vi "Detect QR Code.vi"() -> ()   [LabVIEW 2020, in "examples.lvlib"]
doc: "Demonstrate the QR Code Encoder and the WeChat QR Code Detector."
uses:
  examples.lvlib
  feature_detection/WeChat QR Code Detector/Detection.ctl
  common/Image Points Quad (Float).ctl
  common/Image Point (Float).ctl
  <vilib>/Utility/sysdir.llb/System Directory Type.ctl
  feature_detection/QR Code Encoder/Correction Levels.ctl
  feature_detection/QR Code Encoder/QR Code Encoder.lvclass/QR Code Encoder.ctl
  feature_detection/WeChat QR Code Detector/WeChat QR Code Detector.lvclass/WeChat QR Code Detector.ctl
  image/ARGB Colour.ctl
  feature_detection/QR Code Encoder/Create (Single).vi
  feature_detection/QR Code Encoder/Encode (Single).vi
  image/New Image (ARGB Array).vi
  feature_detection/WeChat QR Code Detector/Detect and Decode Multiple (ARGB).vi
  image/Draw Poly Lines (ARGB).vi
  image/Draw Image to Picture (ARGB).vi
  feature_detection/QR Code Encoder/CreateCore.vi
  feature_detection/QR Code Encoder/EncodeSingleCore.vi
  feature_detection/WeChat QR Code Detector/Detect and Decode Multiple (ARGB).vi/947807d6-cf22-42cc-b024-3c0d53b5d2ed.vi
  image/ARGB Colour to U32 Pixel Value.vi
  image/Draw Poly Lines (ARGB).vi/f4fe866f-059f-471d-887d-2797bd4b3b13.vi
  image/Draw Image to Picture (ARGB).vi/8cd07b1b-062e-4fe4-9e87-2eb3dc89fe0e.vi
  <vilib>/Utility/error.llb/Error Cluster From Error Code.vi
  feature_detection/WeChat QR Code Detector/Create (Model Files Folder).vi
  feature_detection/QR Code Encoder/QR Code Encoder.lvclass
  image/image.lvlib
  feature_detection/WeChat QR Code Detector/WeChat QR Code Detector.lvclass
  common/common.lvlib
panel:
  out "Detections":T1[](array[typedef])
  out "Picture":picture
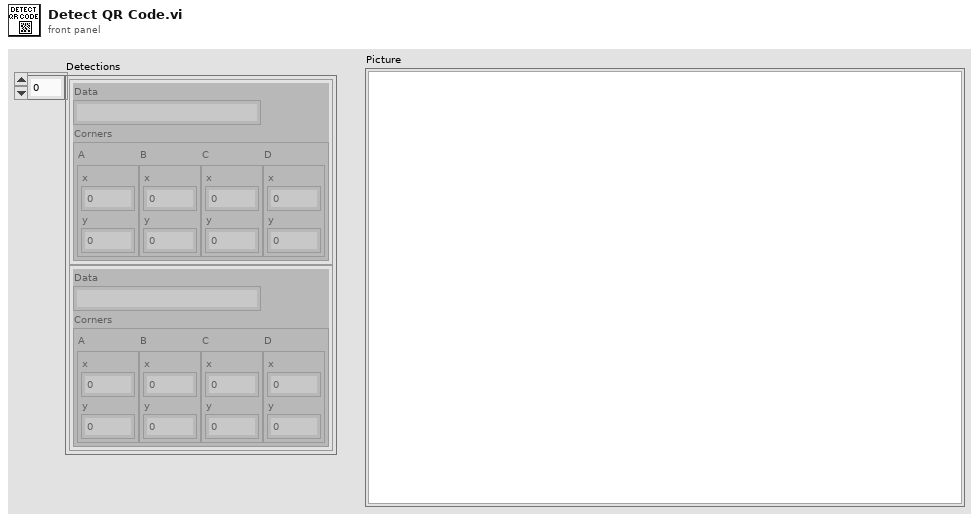
[diagram p1: front panel]
types:
  T1 = typedef "feature_detection.lvlib/WeChat QR Code Detector.lvclass/Detection.ctl" = cluster{"Data":string, "Corners":T2}
  T2 = typedef "common.lvlib/Image Points Quad (Float).ctl" = cluster{"A":T3, "B":T3, "C":T3, "D":T3}
  T3 = typedef "common.lvlib/Image Point (Float).ctl" = cluster{"x":dbl, "y":dbl}
  T4 = typedef "System Directory Type.ctl" = i32
  T5 = typedef "feature_detection.lvlib/QR Code Encoder.lvclass/Correction Levels.ctl" = enum16{"Level L", "Level M", "Level Q", "Level H"}
  T6 = typedef "image.lvlib/ARGB Image.ctl" = refnum<data-value>
  T7 = typedef "image.lvlib/ARGB Colour.ctl" = cluster{"Alpha":u8, "RGB":u32}
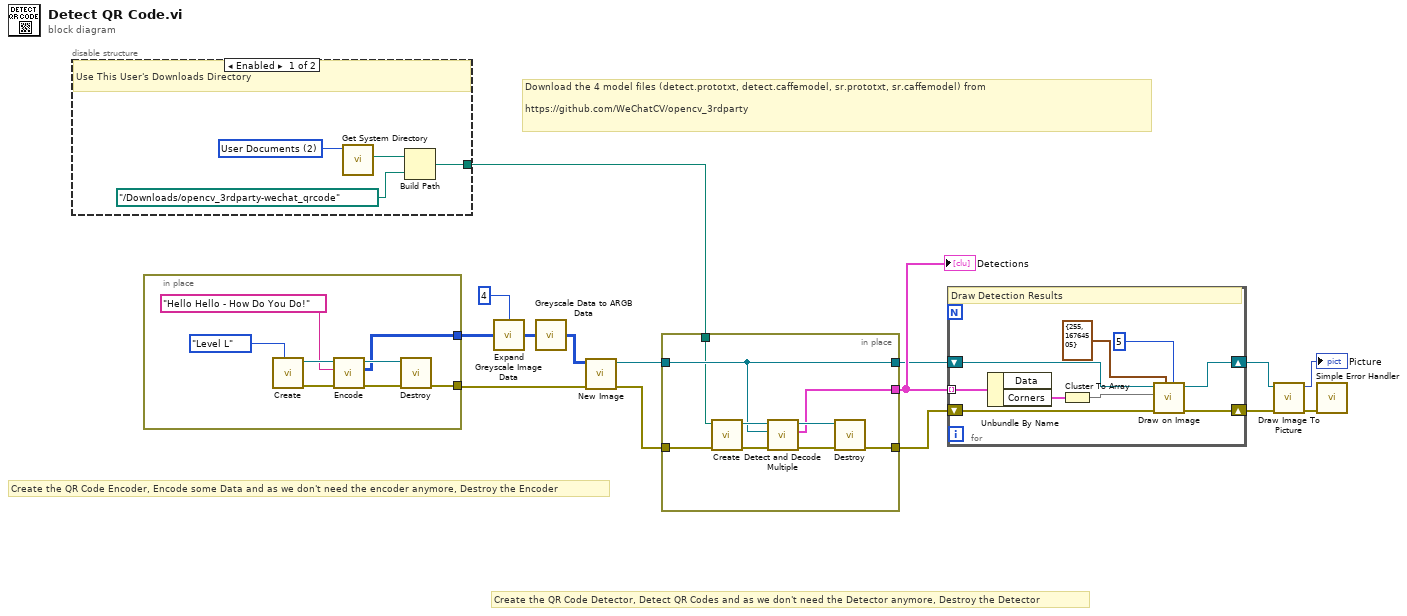
[diagram p0: block diagram]
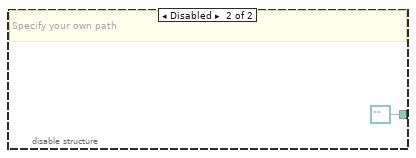
[diagram p2: hidden frame]
diagram:
  # "Download the 4 model files (detect.prototxt, detect.caffemodel, sr.prototxt, sr.caffemodel) from\n \nhttps://github.com/WeChatCV/opencv_3rdparty"
  # "Create the QR Code Detector, Detect QR Codes and as we don't need the Detector anymore, Destroy the Detector"
  # "Create the QR Code Encoder, Encode some Data and as we don't need the encoder anymore, Destroy the Encoder"
  n1 = disable-structure shown="Enabled" {
    disable-tunnel: [w16 path "" ("appended path")] -> w1
    frame Enabled {
      w19 = T4 2 items=["User Home"=0, "User Desktop"=1, "User Documents"=2, "User Application Data"=3, "User Preferences"=4, "User Temporary"=5, "Public Documents"=6, "Public Application Data"=7, "Public Preferences"=8, "Public Cache"=13, "System Core Libraries"=9, "System Installed Libraries"=10, "Application Files"=11, "Boot Volume Root"=12] ("system directory type")
      # "Use This User's Downloads Directory"
      n2 = call <vilib>:"Get System Directory.vi"("system directory type"=w19) -> ("system directory"=w18:path)  [unwired: 10 in]
      n3 = Build Path(base path=w18, name or relative path=path "../Downloads/opencv_3rdparty-wechat_qrcode") -> (appended path=w16:path)
    }
    frame Disabled {
      # "Specify your own path"
    }
  }
  n4 = in-place {
    in-place-border: [w23] -> w6
    in-place-border: [w22] -> w2
    n5 = call-poly "Create.vi"("Correction Level (Default: Level L)"=Correction_Levels."Level L") -> ("error out"=w26:errorcluster, "QR Code Encoder"=w28:refnum<class "QR Code Encoder.lvclass">)  [unwired: 9 in]
    n6 = call-poly "Encode.vi"("error in (no error)"=w26, "Data"="Hello Hello - How Do You Do!", "QR Code Encoder in"=w28) -> ("error out"=w25:errorcluster, "QR Code Image Data"=w23:u8[][], "QR Code Encoder"=w27:refnum<class "QR Code Encoder.lvclass">)  [unwired: 6 in]
    n7 = call "Destroy.vi"("error in (no error)"=w25, "QR Code Encoder in"=w27) -> ("error out"=w22:errorcluster)  [unwired: 9 in]
  }
  n8 = call "Expand Greyscale Image Data.vi"("Greyscale Data"=w6, "Factor"=u16 4) -> ("Expanded Greyscale Data"=w4:u8[][])
  n9 = call "Greyscale Data to ARGB Data.vi"("Greyscale Data"=w4) -> ("ARGB Data"=w5:u32[][])
  n10 = call-poly "New Image.vi"("error in (no error)"=w2, "U32 ARBG Data"=w5) -> ("error out"=w8:errorcluster, "ARGB Image"=w9:T6)  [unwired: 8 in]
  n11 = in-place {
    in-place-border: [w35] -> w15
    in-place-border: [w34] -> w14
    in-place-border: w9 -> [w30]
    in-place-border: w8 -> [w32]
    in-place-border: [w30] -> w7
    in-place-border: w1 -> [w29]
    n12 = call-poly "Create.vi"("error in (no error)"=w32, "Model Files Directory"=w29) -> ("error out"=w31:errorcluster, "WeChat QR Code Detector"=w33:refnum<class "WeChat QR Code Detector.lvclass">)  [unwired: 8 in]
    n13 = call-poly "Detect and Decode Multiple.vi"("error in (no error)"=w31, "ARGB Image in"=w30, "WeChat QR Code Detector in"=w33) -> ("error out"=w36:errorcluster, "Detections"=w35:T1[], "WeChat QR Code Detector"=w37:refnum<class "WeChat QR Code Detector.lvclass">)  [unwired: 6 in]
    n14 = call "Destroy.vi"("error in (no error)"=w36, "WeChat QR Code Detector in"=w37) -> ("error out"=w34:errorcluster)  [unwired: 9 in]
  }
  "Detections" <- w15
  n15 = for {
    shift-right: [w39] -> w12
    shift-left: w7 -> [w46]
    tunnel: w15 -> [w45] mode=indexing
    shift-right: [w42] -> w13
    shift-left: w14 -> [w43]
    # "Draw Detection Results"
    n16 = Unbundle By Name(w45) -> ("Corners"=w44:T2)  [unwired: 1 out]
    n17 = Cluster To Array(cluster=w44) -> (array=w41:T3[])
    n18 = call-poly "Draw on Image.vi"("Thickness (Default: 1)"=5, "ARGB Colour"=T7 {"Alpha"=255, "RGB"=16764505}, "error in (no error)"=w43, "Points"=w41, "ARGB Image in"=w46) -> ("error out"=w42:errorcluster, "ARGB Image"=w39:T6)  [unwired: 5 in]
  }
  n19 = call-poly "Draw Image To Picture.vi"("error in (no error)"=w13, "ARGB Image Source in"=w12) -> ("error out"=w11:errorcluster, "Picture"=→"Picture":picture)  [unwired: 8 in]
  n20 = call <vilib>:"Simple Error Handler.vi"("error in (no error)"=w11) -> ()  [unwired: 4 in, 5 out]
